vi "Delete Top Level.vi"(8 "error in":errorcluster, 9 "Alias":string, 10 "Project Reference":refnum<vi>) -> (0 "error out":errorcluster)   [LabVIEW 2020]
doc: "Removes the TopVI tag from the project."
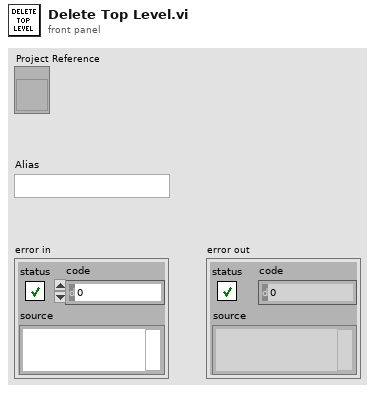
[diagram p1: front panel]
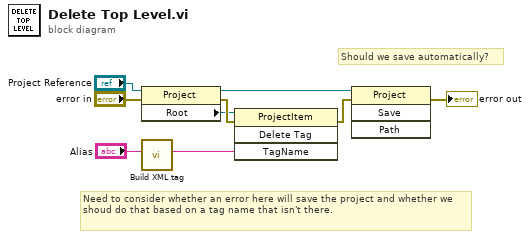
[diagram p0: block diagram]
diagram:
  # "Should we save automatically?"
  # "Need to consider whether an error here will save the project and whether we shoud do that based on a tag name that isn't there."
  n1 = property class="Project"(reference="Project Reference", error in="error in") -> (reference out=w4:refnum<vi>, error out=w7:errorcluster, "Root"=w5:refnum<vi>)
  n2 = call "Build XML tag.vi"("Alias"="Alias") -> ("XML Tag"=w1:string)  [unwired: 10 in]
  n3 = invoke class="ProjectItem" method="Delete Tag"(reference=w5, error in=w7, "TagName"=w1) -> (error out=w6:errorcluster)  [unwired: 1 in, 3 out]
  n4 = invoke class="Project" method="Save"(reference=w4, error in=w6) -> (error out=→"error out":errorcluster)  [unwired: 2 in, 3 out]
